vi "GetSaveBandLevel.vi"(9 "Value in":u16, 11 "Task":enum16{"Read", "Save"}(ring)) -> (1 "Value out":u16)   [LabVIEW 2022 SP3]
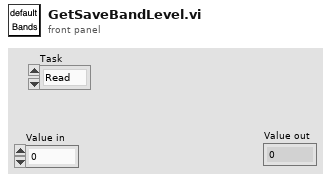
[diagram p1: front panel]
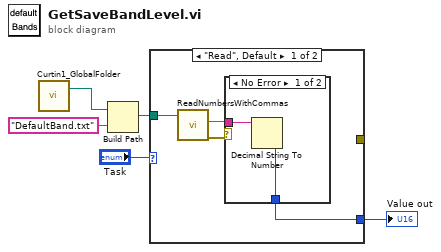
[diagram p0: block diagram]
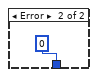
[diagram p2: hidden frame]
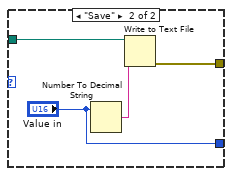
[diagram p3: hidden frame]
diagram:
  n1 = call "Curtin1_GlobalFolder.vi"() -> ("LabVIEW Data Path"=w4:path)  [unwired: 1 in, 1 out]
  n2 = Build Path(base path=w4, name or relative path="DefaultBand.txt") -> (appended path=w2:path)
  n3 = case shown="\"Read\", Default" "Task" {
    tunnel: w2 -> [w6 w16]
    tunnel: [_ w14] -> _
    tunnel: [w9 "Value in"] -> w1
    frame "Read", Default {
      n4 = call "ReadNumbersWithCommas.vi"("file (use dialog)"=w6) -> ("error out"=w8:errorcluster, "text"=w7:string)  [unwired: 7 in, 2 out]
      n5 = case shown="No Error" w8 {
        tunnel: w7 -> [w11 _]
        tunnel: [w10 0] -> w9
        frame No Error {
          n6 = Decimal String To Number(string=w11) -> (number=w10:i32)  [unwired: 2 in, 1 out]
        }
        frame Error {
        }
      }
    }
    frame "Save" {
      n7 = Number To Decimal String(number="Value in") -> (decimal integer string=w15:string)  [unwired: 1 in]
      n8 = Write to Text File(file (use dialog)=w16, text=w15) -> (error out=w14:errorcluster)  [unwired: 2 in, 2 out]
    }
  }
  "Value out" <- w1
